vi "test-linear-filter-get-pulse-data.vi"(11 "T":dbl) -> (3 "Output":dbl)   [LabVIEW 2019]
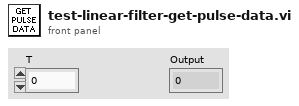
[diagram p1: front panel]
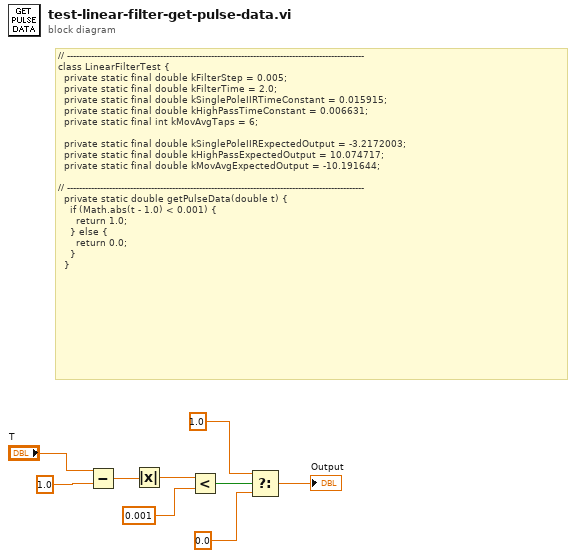
[diagram p0: block diagram]
diagram:
  # "// ---------------------------------------------------------------------------------------------------\nclass LinearFilterTest {\n  private static final double kFilterStep = 0.005;\n  private static final double kFilterTime = 2.0;\n  private static final double kSinglePoleIIRTimeConstant = 0.015915;\n  private static final double kHighPassTimeConstant = 0.006631;\n  private static final int kMovAvgTaps = 6;\n\n  private static final double kSinglePoleIIRExpectedOutput = -3.2172003;\n  private static final double kHighPassExpectedOutput = 10.074717;\n  private static final double kMovAvgExpectedOutput = -10.191644;\n\n// ---------------------------------------------------------------------------------------------------\n  private static double getPulseData(double t) {\n    if (Math.abs(t - 1.0) < 0.001) {\n      return 1.0;\n    } else {\n      return 0.0;\n    }\n  }"
  n1 = Subtract(x="T", y=1.0) -> (x-y=w7:dbl)
  n2 = Absolute Value(x=w7) -> (abs(x)=w6:dbl)
  n3 = Less?(x=w6, y=0.001) -> (x < y?=w4:bool)
  n4 = Select(t=1.0, s=w4, f=0.0) -> (s? t:f=→"Output":dbl)
